vi "Rename Node.vi"(0 "FSM.Graph In":refnum<class "FSM.Graph.lvclass">, 7 "Index":i32, 9 "New name":string) -> (4 "FSM.Graph Out":refnum<class "FSM.Graph.lvclass">)   [LabVIEW 2020, in "FSM.Graph.lvclass"]
uses:
  FSM.Graph.lvclass
  FSM.Graph.lvclass/FSM.Graph.ctl
  FSM.Node/FSM.Node.lvclass/FSM.Node.ctl
  FSM.Node/Read Name.vi
  FSM.Node/FSM.Node.lvclass
  FSM.Edge/FSM.Edge.lvclass
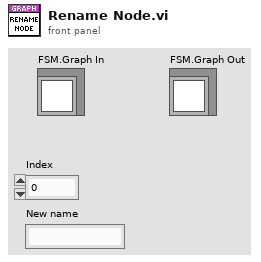
[diagram p1: front panel]
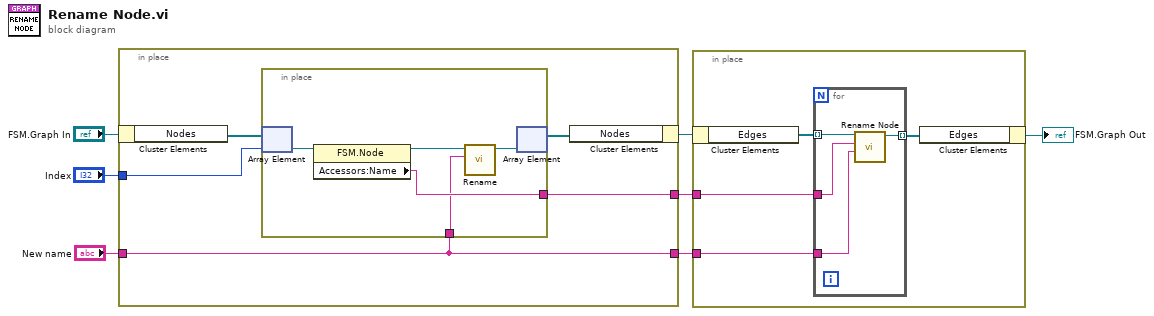
[diagram p0: block diagram]
diagram:
  n1 = in-place {
    in-place-border: "Index" -> [w11]
    in-place-border: "New name" -> [w8]
    in-place-border: [w9] -> w3
    in-place-border: [w8] -> w2
    n2 = in-place-cluster #1("FSM.Graph In") -> ("Nodes"=w12:refnum<class "FSM.Node.lvclass">[])
    n3 = in-place {
      in-place-border: w8 -> [w13]
      in-place-border: [w16] -> w9
      n4 = in-place-array #2(w12, w11) -> (w17:refnum<class "FSM.Node.lvclass">)
      n5 = property class="FSM.Node"(reference=w17) -> (reference out=w15:refnum<class "FSM.Node.lvclass">, "Accessors:Name"=w16:string)  [unwired: 1 in, 1 out]
      n6 = call "Rename.vi"("Name"=w13, "FSM in"=w15) -> ("FSM out"=w14:refnum<class "FSM.Node.lvclass">)  [unwired: 8 in, 1 out]
      n7 = in-place-array #2(w14) -> (w10:refnum<class "FSM.Node.lvclass">[])  [unwired: 1 out]
    }
    n8 = in-place-cluster #1("Nodes"=w10) -> (w4:refnum<class "FSM.Graph.lvclass">)
  }
  n9 = in-place {
    in-place-border: w3 -> [w19]
    in-place-border: w2 -> [w20]
    n10 = in-place-cluster #3(w4) -> ("Edges"=w21:refnum<class "FSM.Edge.lvclass">[])
    n11 = for {
      tunnel: w21 -> [w25] mode=indexing
      tunnel: w20 -> [w23]
      tunnel: w19 -> [w24]
      tunnel: [w22] -> w18 mode=indexing
      n12 = call "Rename Node.vi"("New Name"=w23, "Old Name"=w24, "FSM.Edge in"=w25) -> ("FSM.Edge out"=w22:refnum<class "FSM.Edge.lvclass">)  [unwired: 7 in, 1 out]
    }
    n13 = in-place-cluster #3("Edges"=w18) -> (→"FSM.Graph Out":refnum<class "FSM.Graph.lvclass">)
  }
